vi "Read Array of Motor Objs.vi"(11 "Motions in":refnum<class "Motions.lvclass">) -> (2 "Array of Motor Objs":refnum<class "Motor.lvclass">[](array[class]), 3 "Motions out":refnum<class "Motions.lvclass">)   [LabVIEW 2016, in "Hardware.lvlib" / "Motions.lvlib" / "Motions.lvclass"]
uses:
  <userlib>/Common Components/Hardware/Abstract System/Motions/Motions/Motions.lvclass
  <userlib>/Common Components/Hardware/Motor/Motor/Motor.lvclass
  <userlib>/Common Components/Hardware/Abstract System/Motions/Motions/Motions.lvclass/Motions.ctl
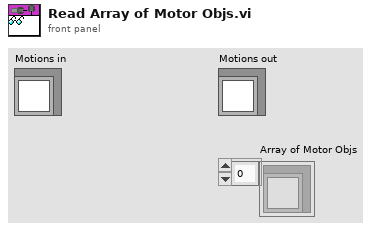
[diagram p1: front panel]
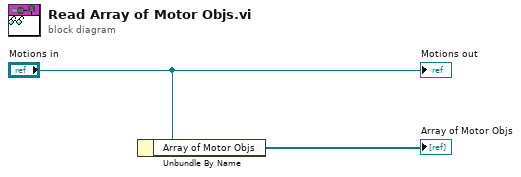
[diagram p0: block diagram]
diagram:
  n1 = Unbundle By Name("Motions in") -> ("Array of Motor Objs"=→"Array of Motor Objs":refnum<class "Motor.lvclass">[])
  "Motions out" <- "Motions in"
